vi "Mouse Click Event.vi"(8 "错误输入（无错误）":errorcluster, 11 "Mouse Click":T1) -> (0 "错误输出":errorcluster)   [LabVIEW 2012, in "API.lvlib"]
uses:
  API.lvlib
  Mouse_Click.ctl
  Mouse_Event.ctl
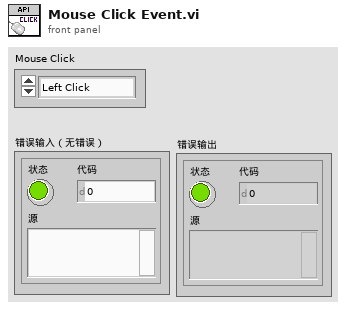
[diagram p1: front panel]
types:
  T1 = typedef "API.lvlib/Mouse_Click.ctl" = enum16{"Left Click", "Left dbClick", "Right Click", "Right dbClick", "Middle Click", "Middle dbClick"}
  T2 = typedef "API.lvlib/Mouse_Event.ctl" = u32
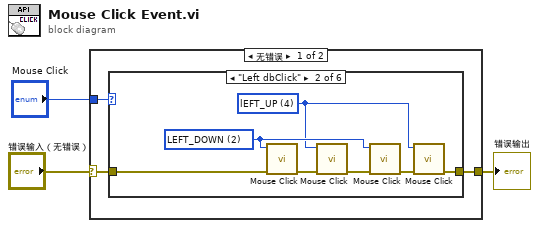
[diagram p0: block diagram]
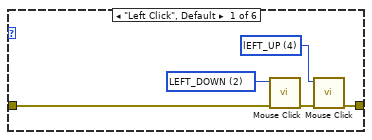
[diagram p2: hidden frame]
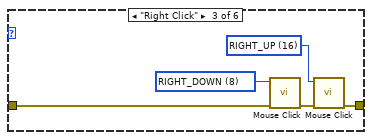
[diagram p3: hidden frame]
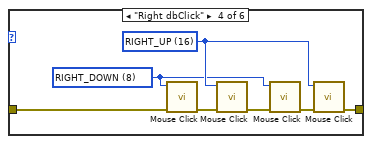
[diagram p4: hidden frame]
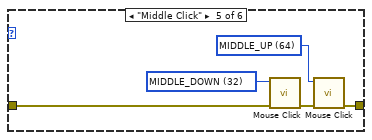
[diagram p5: hidden frame]
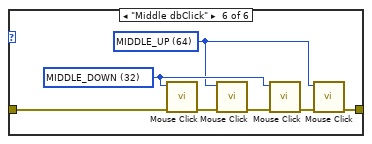
[diagram p6: hidden frame]
diagram:
  n1 = case shown="无错误" "错误输入（无错误）" {
    selector: "错误输入（无错误）" -> [w5 w43]
    tunnel: [w6 w43] -> w3
    tunnel: "Mouse Click" -> [w4 _]
    frame No Error {
      n2 = case shown="\"Left dbClick\"" w4 {
        tunnel: w5 -> [w11 w18 w23 w29 w35 w42]
        tunnel: [w8 w14 w21 w26 w31 w38] -> w6
        frame "Left Click", Default {
          w7 = T2 4 items=["MOVE"=1, "LEFT_DOWN"=2, "lEFT_UP"=4, "RIGHT_DOWN"=8, "RIGHT_UP"=16, "MIDDLE_DOWN"=32, "MIDDLE_UP"=64, "MOUSE_WHEEL"=128, "ABSOLUTE"=32768] ("文本下拉列表")
          w10 = T2 2 items=["MOVE"=1, "LEFT_DOWN"=2, "lEFT_UP"=4, "RIGHT_DOWN"=8, "RIGHT_UP"=16, "MIDDLE_DOWN"=32, "MIDDLE_UP"=64, "MOUSE_WHEEL"=128, "ABSOLUTE"=32768] ("文本下拉列表")
          n3 = call "Mouse Click.vi"("错误输入（无错误）"=w11, "鼠标操作"=w10) -> ("错误输出"=w9:errorcluster)  [unwired: 9 in]
          n4 = call "Mouse Click.vi"("错误输入（无错误）"=w9, "鼠标操作"=w7) -> ("错误输出"=w8:errorcluster)  [unwired: 9 in]
        }
        frame "Left dbClick" {
          w12 = T2 4 items=["MOVE"=1, "LEFT_DOWN"=2, "lEFT_UP"=4, "RIGHT_DOWN"=8, "RIGHT_UP"=16, "MIDDLE_DOWN"=32, "MIDDLE_UP"=64, "MOUSE_WHEEL"=128, "ABSOLUTE"=32768] ("文本下拉列表")
          w13 = T2 2 items=["MOVE"=1, "LEFT_DOWN"=2, "lEFT_UP"=4, "RIGHT_DOWN"=8, "RIGHT_UP"=16, "MIDDLE_DOWN"=32, "MIDDLE_UP"=64, "MOUSE_WHEEL"=128, "ABSOLUTE"=32768] ("文本下拉列表")
          n5 = call "Mouse Click.vi"("错误输入（无错误）"=w18, "鼠标操作"=w13) -> ("错误输出"=w17:errorcluster)  [unwired: 9 in]
          n6 = call "Mouse Click.vi"("错误输入（无错误）"=w17, "鼠标操作"=w12) -> ("错误输出"=w16:errorcluster)  [unwired: 9 in]
          n7 = call "Mouse Click.vi"("错误输入（无错误）"=w16, "鼠标操作"=w13) -> ("错误输出"=w15:errorcluster)  [unwired: 9 in]
          n8 = call "Mouse Click.vi"("错误输入（无错误）"=w15, "鼠标操作"=w12) -> ("错误输出"=w14:errorcluster)  [unwired: 9 in]
        }
        frame "Right Click" {
          w19 = T2 16 items=["MOVE"=1, "LEFT_DOWN"=2, "lEFT_UP"=4, "RIGHT_DOWN"=8, "RIGHT_UP"=16, "MIDDLE_DOWN"=32, "MIDDLE_UP"=64, "MOUSE_WHEEL"=128, "ABSOLUTE"=32768] ("文本下拉列表")
          w20 = T2 8 items=["MOVE"=1, "LEFT_DOWN"=2, "lEFT_UP"=4, "RIGHT_DOWN"=8, "RIGHT_UP"=16, "MIDDLE_DOWN"=32, "MIDDLE_UP"=64, "MOUSE_WHEEL"=128, "ABSOLUTE"=32768] ("文本下拉列表")
          n9 = call "Mouse Click.vi"("错误输入（无错误）"=w23, "鼠标操作"=w20) -> ("错误输出"=w22:errorcluster)  [unwired: 9 in]
          n10 = call "Mouse Click.vi"("错误输入（无错误）"=w22, "鼠标操作"=w19) -> ("错误输出"=w21:errorcluster)  [unwired: 9 in]
        }
        frame "Right dbClick" {
          w25 = T2 16 items=["MOVE"=1, "LEFT_DOWN"=2, "lEFT_UP"=4, "RIGHT_DOWN"=8, "RIGHT_UP"=16, "MIDDLE_DOWN"=32, "MIDDLE_UP"=64, "MOUSE_WHEEL"=128, "ABSOLUTE"=32768] ("文本下拉列表")
          w24 = T2 8 items=["MOVE"=1, "LEFT_DOWN"=2, "lEFT_UP"=4, "RIGHT_DOWN"=8, "RIGHT_UP"=16, "MIDDLE_DOWN"=32, "MIDDLE_UP"=64, "MOUSE_WHEEL"=128, "ABSOLUTE"=32768] ("文本下拉列表")
          n11 = call "Mouse Click.vi"("错误输入（无错误）"=w29, "鼠标操作"=w24) -> ("错误输出"=w28:errorcluster)  [unwired: 9 in]
          n12 = call "Mouse Click.vi"("错误输入（无错误）"=w28, "鼠标操作"=w25) -> ("错误输出"=w30:errorcluster)  [unwired: 9 in]
          n13 = call "Mouse Click.vi"("错误输入（无错误）"=w30, "鼠标操作"=w24) -> ("错误输出"=w27:errorcluster)  [unwired: 9 in]
          n14 = call "Mouse Click.vi"("错误输入（无错误）"=w27, "鼠标操作"=w25) -> ("错误输出"=w26:errorcluster)  [unwired: 9 in]
        }
        frame "Middle Click" {
          w32 = T2 64 items=["MOVE"=1, "LEFT_DOWN"=2, "lEFT_UP"=4, "RIGHT_DOWN"=8, "RIGHT_UP"=16, "MIDDLE_DOWN"=32, "MIDDLE_UP"=64, "MOUSE_WHEEL"=128, "ABSOLUTE"=32768] ("文本下拉列表")
          w33 = T2 32 items=["MOVE"=1, "LEFT_DOWN"=2, "lEFT_UP"=4, "RIGHT_DOWN"=8, "RIGHT_UP"=16, "MIDDLE_DOWN"=32, "MIDDLE_UP"=64, "MOUSE_WHEEL"=128, "ABSOLUTE"=32768] ("文本下拉列表")
          n15 = call "Mouse Click.vi"("错误输入（无错误）"=w35, "鼠标操作"=w33) -> ("错误输出"=w34:errorcluster)  [unwired: 9 in]
          n16 = call "Mouse Click.vi"("错误输入（无错误）"=w34, "鼠标操作"=w32) -> ("错误输出"=w31:errorcluster)  [unwired: 9 in]
        }
        frame "Middle dbClick" {
          w36 = T2 64 items=["MOVE"=1, "LEFT_DOWN"=2, "lEFT_UP"=4, "RIGHT_DOWN"=8, "RIGHT_UP"=16, "MIDDLE_DOWN"=32, "MIDDLE_UP"=64, "MOUSE_WHEEL"=128, "ABSOLUTE"=32768] ("文本下拉列表")
          w37 = T2 32 items=["MOVE"=1, "LEFT_DOWN"=2, "lEFT_UP"=4, "RIGHT_DOWN"=8, "RIGHT_UP"=16, "MIDDLE_DOWN"=32, "MIDDLE_UP"=64, "MOUSE_WHEEL"=128, "ABSOLUTE"=32768] ("文本下拉列表")
          n17 = call "Mouse Click.vi"("错误输入（无错误）"=w42, "鼠标操作"=w37) -> ("错误输出"=w41:errorcluster)  [unwired: 9 in]
          n18 = call "Mouse Click.vi"("错误输入（无错误）"=w41, "鼠标操作"=w36) -> ("错误输出"=w40:errorcluster)  [unwired: 9 in]
          n19 = call "Mouse Click.vi"("错误输入（无错误）"=w40, "鼠标操作"=w37) -> ("错误输出"=w39:errorcluster)  [unwired: 9 in]
          n20 = call "Mouse Click.vi"("错误输入（无错误）"=w39, "鼠标操作"=w36) -> ("错误输出"=w38:errorcluster)  [unwired: 9 in]
        }
      }
    }
    frame Error {
    }
  }
  "错误输出" <- w3
